vi "tree_control_parameters.vi"(10 "Point":T1, 11 "Parameters Tree":refnum<vi>) -> ()   [LabVIEW 2019]
uses:
  <vilib>/Utility/miscctls.llb/LVPositionTypeDef.ctl
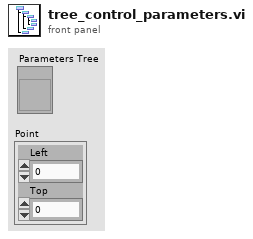
[diagram p1: front panel]
types:
  T1 = typedef "LVPositionTypeDef.ctl" = cluster{"Left":i32, "Top":i32}
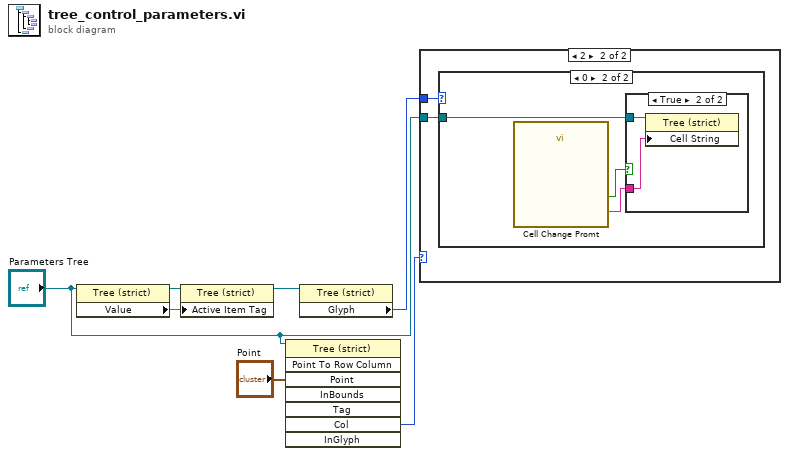
[diagram p0: block diagram]
diagram:
  n1 = property on="Property Node" class="Tree (strict)"(reference="Parameters Tree") -> (reference out=w7:refnum<vi>, "Value"=w5:string)  [unwired: 1 in, 1 out]
  n2 = property on="Property Node" class="Tree (strict)"(reference=w7, "Active Item Tag"=w5) -> (reference out=w6:refnum<vi>)  [unwired: 1 in, 1 out]
  n3 = invoke on="Invoke Node" class="Tree (strict)" method="Point To Row Column"(reference="Parameters Tree", "Point"="Point") -> ("Col"=w4:i32)  [unwired: 6 in, 7 out]
  n4 = property class="Tree (strict)"(reference=w6) -> ("Glyph"=w3:i32)  [unwired: 1 in, 2 out]
  n5 = case shown="2" w4 {
    tunnel: "Parameters Tree" -> [_ w9]
    tunnel: w3 -> [_ w8]
    frame 0, 1, Default {
    }
    frame 2 {
      n6 = case shown="0" w8 {
        tunnel: w9 -> [_ w11]
        frame 15, Default {
        }
        frame 0 {
          n7 = call "Cell Change Promt"() -> ("New Value"=w12:string, "OK"=w10:bool)  [unwired: 17 in, 1 out]
          n8 = case shown="True" w10 {
            tunnel: w12 -> [_ w14]
            tunnel: w11 -> [_ w13]
            frame False {
            }
            frame True {
              n9 = property class="Tree (strict)"(reference=w13, "Cell String"=w14) -> ()  [unwired: 1 in, 2 out]
            }
          }
        }
      }
    }
  }
